vi "daq_example_stimulate_from_file.vi"() -> ()   [LabVIEW 2015]
uses:
  <vilib>/Platform/storage/lvStorage.llb/_openFunction.ctl
  <vilib>/DAQmx/write.llb/DAQmx Write (Analog Wfm 1Chan NSamp).vi
  <vilib>/DAQmx/create/channels.llb/DAQmx Create Channel (AO-Voltage-Basic).vi
  <vilib>/DAQmx/configure/timing.llb/DAQmx Timing (Sample Clock).vi
  <vilib>/Platform/storage/lvStorage.llb/_openStorageWithRootAutoDetect.vi
  <vilib>/Platform/storage/lvStorage.llb/xStorage/xStorageSupp/ErrorOut.vi
  <vilib>/Platform/storage/lvStorage.llb/_queryPropPoly.vi
  <vilib>/Platform/storage/lvStorage.llb/_queryPropString.vi
  <vilib>/Platform/storage/lvStorage.llb/_queryGenericObjects.vi
  <vilib>/Platform/storage/lvStorage.llb/_loadAllDdt.vi
  <vilib>/DAQmx/miscellaneous.llb/DAQmx Fill In Error Info.vi
  <vilib>/Platform/storage/lvStorage.llb/xStorage/Open Data Storage/Open Data Storage.xnode
  <vilib>/Platform/storage/lvStorage.llb/xStorage/Read Data/Read Data.xnode
  <resource>/objmgr/daqmx.rc
panel:
  out "Waveform Graph":dynamicdata(graph)
  out "DataPlugin name out":string
  in  "Path":path=path "E:/code/labview-phys-io/001_pure_sines_151013_10Hz.mat"
  out "Actual Sample Rate":dbl=1000.0 format="%0.2f"
  out "Numeric":dbl
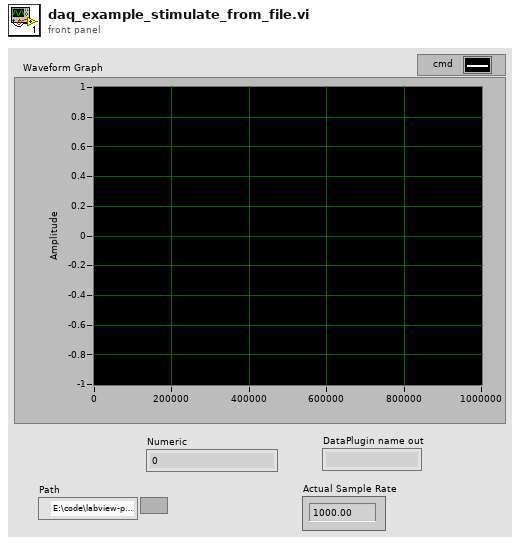
[diagram p1: front panel]
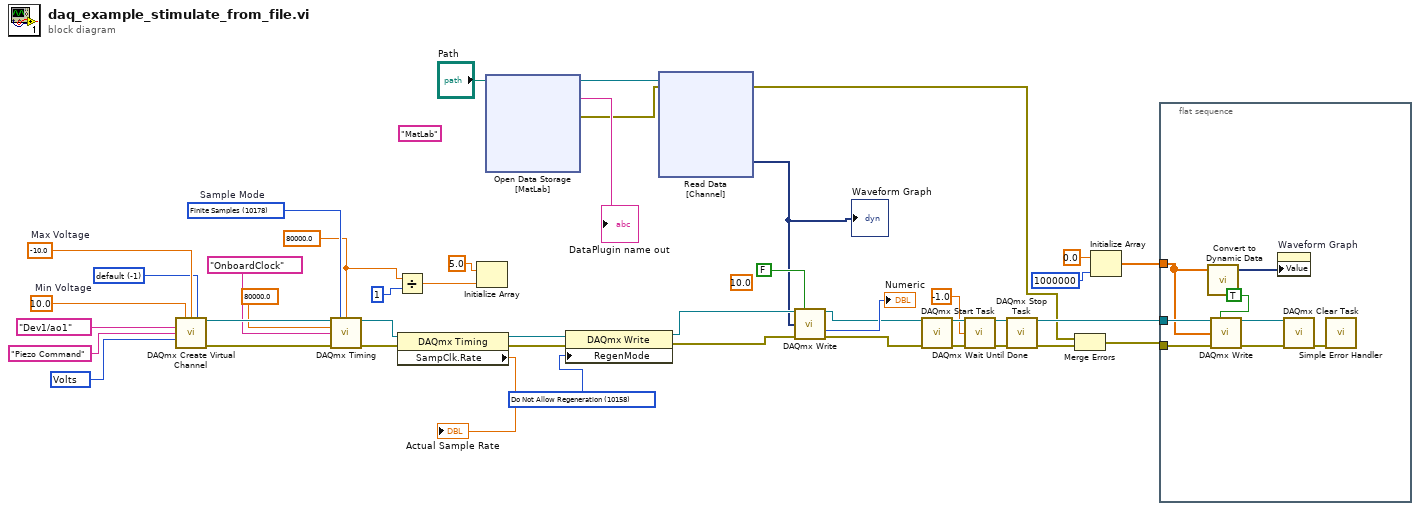
[diagram p0: block diagram]
diagram:
  (unwired) "MatLab"
  w13 = 10158 items=["Allow Regeneration"=10097, "Do Not Allow Regeneration"=10158] ("RegenMode")
  w22 = 80000.0
  (unwired) 10.0
  w35 = 10178 items=["Finite Samples"=10178, "Continuous Samples"=10123, "Hardware Timed Single Point"=12522]  # Sample Mode
  w36 = -1 items=["default"=-1, "RSE"=10083, "NRSE"=10078, "Differential"=10106, "Pseudodifferential"=12529] ("input terminal configuration")
  w37 = 10348 items=["Volts"=10348, "From Custom Scale"=10065] ("units")
  w41 = 10.0  # Min Voltage
  w40 = -10.0  # Max Voltage
  n1 = call-poly <vilib>:"DAQmx Create Virtual Channel.vi"("maximum value"=w41, "minimum value"=w40, "output terminal configuration"=w36, "physical channels"=tag "Dev1/ao1" ("DAQmx Physical Channel"), "name to assign"="Piezo Command", "units"=w37) -> ("task out"=w43:refnum<k21>, "error out"=w44:errorcluster)  [unwired: 8 in]
  n2 = call-poly <vilib>:"DAQmx Timing.vi"("task/channels in"=w43, "sample mode"=w35, "samples per channel"=w22, "rate"=80000.0, "source"=tag "OnboardClock" ("Sample Clock Source"), "error in"=w44) -> ("task out"=w33:refnum<k21>, "error out"=w32:errorcluster)  [unwired: 8 in]
  n3 = Divide(x=w22, y=1) -> (x/y=w21:dbl)
  n4 = property class="DAQmx Timing"(reference=w33, error in=w32) -> (reference out=w19:refnum<k21>, error out=w18:errorcluster, "SampClk.Rate"=→"Actual Sample Rate":dbl)
  n5 = Initialize Array(5.0 ("element"), w21) -> ()  [unwired: 1 out]
  n6 = xnode "Open Data Storage\n[MatLab]"("file path"="Path") -> ("storage refnum (file)"=w10:refnum<k20>, "DataPlugin name out"=→"DataPlugin name out":string, "error out"=w4:errorcluster)  [unwired: 4 in]
  n7 = property class="DAQmx Write"(reference=w19, error in=w18, "RegenMode"=w13) -> (reference out=w17:refnum<k21>, error out=w16:errorcluster)
  n8 = xnode "Read Data\n[Channel]"("storage refnum (file)"=w10, "error in"=w4) -> ("Signal"=w8:dynamicdata, "error out"=w3:errorcluster)  [unwired: 2 in, 2 out]
  "Waveform Graph" <- w8
  n9 = call-poly <vilib>:"DAQmx Write.vi"("task/channels in"=w17, "auto start"=FALSE, "data"=w8, "error in"=w16) -> ("task out"=w14:refnum<k21>, "number of samples written per channel"=→"Numeric":u32, "error out"=w15:errorcluster)  [unwired: 9 in]
  n10 = call <vilib>:"DAQmx Start Task.vi"("task/channels in"=w14, "error in"=w15) -> ("task out"=w26:refnum<k21>, "error out"=w27:errorcluster)  [unwired: 12 in]
  n11 = call <vilib>:"DAQmx Wait Until Done.vi"("task/channels in"=w26, "timeout (sec)"=-1.0, "error in"=w27) -> ("task out"=w29:refnum<k21>, "error out"=w28:errorcluster)  [unwired: 11 in]
  n12 = call <vilib>:"DAQmx Stop Task.vi"("task/channels in"=w29, "error in"=w28) -> ("task out"=w12:refnum<k21>, "error out"=w1:errorcluster)  [unwired: 12 in]
  n13 = Merge Errors(w3, w1) -> (w2:errorcluster)
  n14 = Initialize Array(0.0 ("element"), 1000000 ("dimension size")) -> (w5:dbl[])
  n15 = flat-sequence {
    tunnel: w12 -> [w48]
    tunnel: w2 -> [w47]
    tunnel: w5 -> [w45]
    frame #0 {
      n16 = call "Convert to Dynamic Data"("Array"=w45) -> ("Dynamic Data Type"=w46:dynamicdata)  [unwired: 3 in]
      n17 = call-poly <vilib>:"DAQmx Write.vi"("task/channels in"=w48, "auto start"=TRUE, "data"=w45, "error in"=w47) -> ("task out"=w51:refnum<k21>, "error out"=w50:errorcluster)  [unwired: 9 in, 1 out]
      n18 = property on="Waveform Graph" class="WFGraph (strict)"("Value"=w46) -> ()  [unwired: 2 in, 2 out]
      n19 = call <vilib>:"DAQmx Clear Task.vi"("task in"=w51, "error in"=w50) -> ("error out"=w52:errorcluster)  [unwired: 13 in]
      n20 = call <vilib>:"Simple Error Handler.vi"("error in (no error)"=w52) -> ()  [unwired: 4 in, 5 out]
    }
  }
